vi "zadanie_3.vi"() -> ()   [LabVIEW 2020]
panel:
  out "indeks (max)":dbl[](array[numeric])
  out "indeks (min)":dbl[](array[numeric])
  in  "stop":bool
  out "min wartosc":dbl
  out "max  wartosc":dbl
  out "liczba kolumn":dbl
  out "liczba wierszy":dbl
  in  "zwroc minimalna i maksymalna wartosc":bool
  in  "sprawdz wymiar tablicy":bool
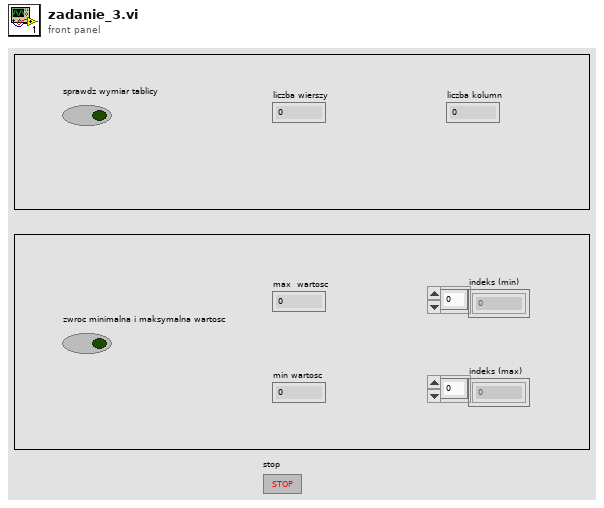
[diagram p1: front panel]
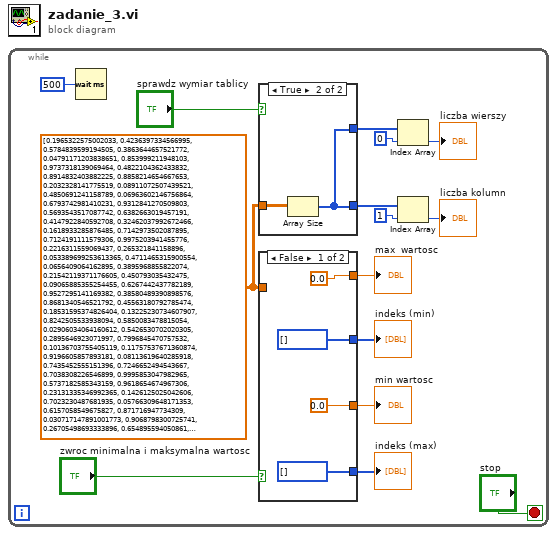
[diagram p0: block diagram]
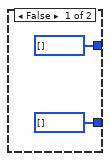
[diagram p2: hidden frame]
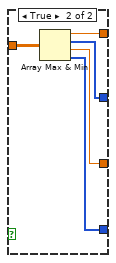
[diagram p3: hidden frame]
diagram:
  n1 = while {
    stop <- "stop" stop-if-true
    w7 = dbl[][] [[0.1965322575002033, 0.4236397334566995, 0.5784839599194505, 0.3863644657521772, 0.04791171203838651, 0.853999211948103], [0.9737318139069464, 0.4822104362433832, 0.8914832403882225, 0.8858214654667653, 0.2032328141775519, 0.08911072507439521], [0.4850691241158789, 0.06963602146756864, 0.6793742981410231, 0.9312841270509803, 0.5693543517087742, 0.6382663019457191], [0.4147922840592708, 0.32462037992672466, 0.1618933285876485, 0.7142973502087895, 0.7124191111579306, 0.9975203941455776], [0.2216311559069437, 0.265321841158896, 0.053389699253613365, 0.4711465315900554, 0.0656409064162895, 0.3895968855822074], [0.21542119371176605, 0.450793035432475, 0.09065885355254455, 0.6267442437782189, 0.9527295141169382, 0.38580489390898576], [0.8681340546521792, 0.45563180792785474, 0.18531595374826404, 0.13225230734607907, 0.8242505533938094, 0.5850083478815054], [0.02906034064160612, 0.5426530702020305, 0.2895646923071997, 0.7996845470757532, 0.10136703755405119, 0.11757537671360874], [0.9196605857893181, 0.08113619640285918, 0.7435452555151396, 0.7246652494543667, 0.7038308226546899, 0.9995853047982965], [0.5737182585343159, 0.9618654674967306, 0.23131335346992365, 0.1426125025042606, 0.7023230487681935, 0.05766309648171353], [0.6157058549675827, 0.871716947734309, 0.030717147891001773, 0.9068798300725741, 0.26705498693333896, 0.654895594050861], [0.7894320550775396, 0.8442090964572024, 0.6866090374135262, 0.37274667477768997, 0.7517140421486013, 0.19692790116554582]] ("Array")
    n2 = Wait (ms)(milliseconds to wait=u32 500) -> ()  [unwired: 1 out]
    n3 = case shown="True" "sprawdz wymiar tablicy" {
      tunnel: w7 -> [_ w19]
      tunnel: [i32[] [] w18] -> w6
      tunnel: [i32[] [] w18] -> w3
      frame False {
      }
      frame True {
        n4 = Array Size(array=w19) -> (size(s)=w18:i32[])
      }
    }
    n5 = case shown="False" "zwroc minimalna i maksymalna wartosc" {
      tunnel: [0.0 w28] -> w13
      tunnel: [0.0 w27] -> w12
      tunnel: w7 -> [_ w26]
      tunnel: [i32[] [] w25] -> w11
      tunnel: [i32[] [] w24] -> w10
      frame False {
      }
      frame True {
        n6 = Array Max & Min(array=w26) -> (max value=w28:dbl, max index (indices)=w25:i32[], min value=w27:dbl, min index (indices)=w24:i32[])
      }
    }
    "max  wartosc" <- w13
    "min wartosc" <- w12
    "indeks (min)" <- w11
    "indeks (max)" <- w10
    n7 = Index Array(array=w6, index=0) -> (element=→"liczba wierszy":i32)
    n8 = Index Array(array=w3, index=1) -> (element=→"liczba kolumn":i32)
  }
